vi "DDL.vi"(0 "System no.":i32=1 min=1 max=4 step=1, 2 "Table no.":i32=1, 3 "Offset":i32, 4 "No.of digits":i16=6, 5 "error in":errorcluster, 6 "Values":dbl[](array[numeric]) format="%.6f") -> (19 "error out":errorcluster)   [LabVIEW 2020]
doc: "Loads the specified values to the specified DDL table. Please refer to the controller user manual for units and restrictions.\n\nE-710: Table number can be 1 to 8. First stored value in table has index 1, index 0 must be DDL repeat number. Maximum 32768 values can be stored.\n\nE-712: Table number can be 1 to the maximum number of axes (query with TLT? for the number of DDL tables). First stored value in table has index 1, so Offset must be greater than zero. Maximum 262,144 values can be stored. Due to the maximum numbers of parameters per command only 30 DDL table values can be set per one command call.\n\nE-725, E-727: Table number can be 1 to the maximum number of axes (query with TLT? for the number of DDL tables). First stored value in table has index 1, so Offset must be greater than zero. Maximum 262,144 values can be stored. Due to the maximum numbers of parameters per command only 30 DDL table values can be set per one command call.\n\nE-753: Table number can be 1. First stored value in table has index 1, so Offset must be greater than zero. Maximum 65,536 values can be stored. Due to the maximum numbers of parameters per command only 30 DDL table values can be set per one command call.\n\nE-754: Table number can be 1. First stored value in table has index 1, so Offset must be greater than zero. Maximum 1,046,076 values can be stored. Due to the maximum numbers of parameters per command only 30 DDL table values can be set per one command call."
uses:
  General command.llb/Controller names.ctl
  General command.llb/Global2 (Array).vi
panel:
  # "Loads the specified values to the specified DDL Table. Please refer to \nthe User Manual for units and restrictions."
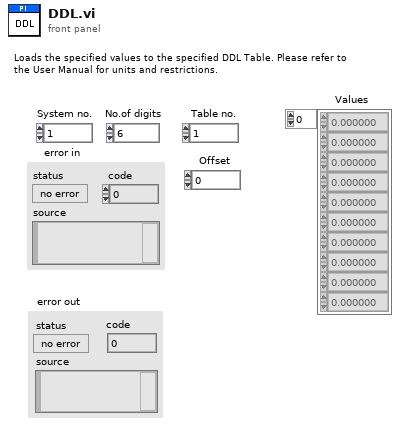
[diagram p1: front panel]
types:
  T1 = typedef "Controller names.ctl" = enum16{"None", "Analog", "C-702", "C-413", "C-414", "C-843", "C-843.PM", "C-844", "C-848", "C-865", "C-866", "C-867", "C-877", "C-880", "C-884", "C-885", "C-886", "C-887", "C-891", "E-135", "E-516", "E-517", "E-518", "E-709", "E-710", "E-712", "E-725", "E-727", "E-753", "E-754", "E-755", "E-761", "E-816", "E-861", "E-870", "E-871", "E-872", "E-873", "E-874", "F-206", "HydraPollux", "M-840", "M-850", "M-8X0", "Mercury", "Mercury_GCS", "PI_GCS2"}
  T2 = cluster{"Conn. axes":string[], "Controller name":T1}[]
  T3 = cluster{"Conn. axes":string[], "Controller name":T1}
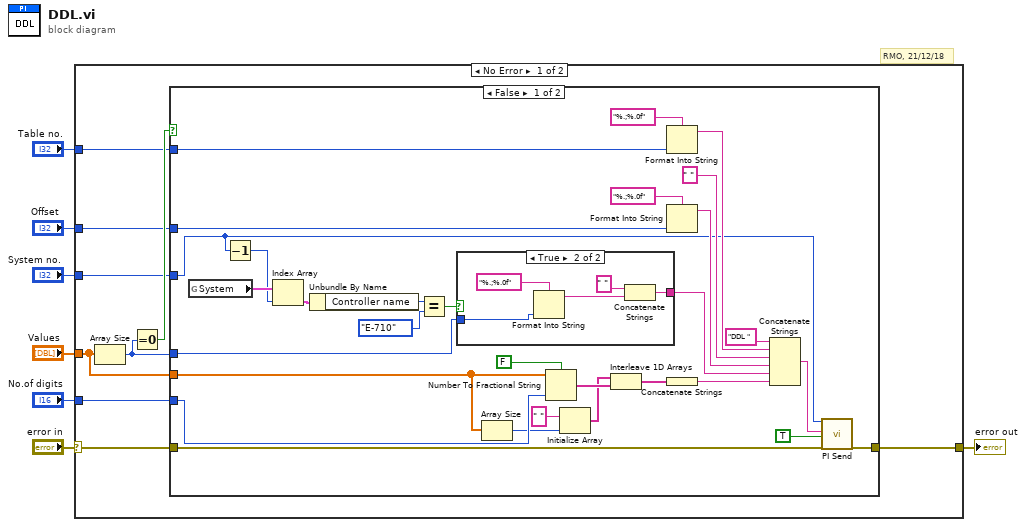
[diagram p0: block diagram]
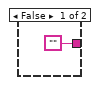
[diagram p2: hidden frame]
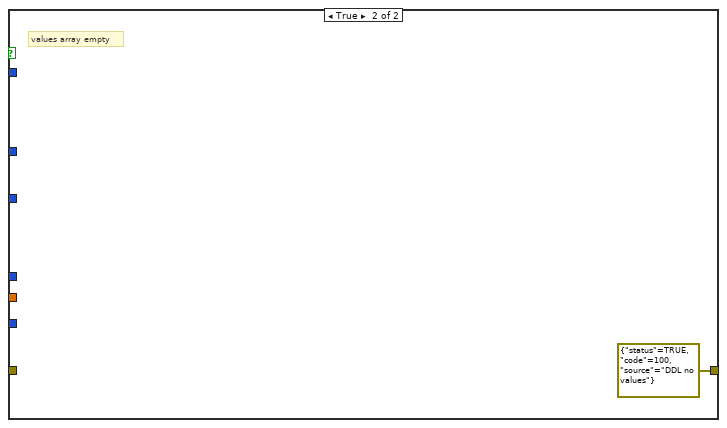
[diagram p3: hidden frame]
diagram:
  # "RMO, 21/12/18"
  n1 = case shown="No Error" "error in" {
    selector: "error in" -> [w13 w54]
    tunnel: [w16 w54] -> w7
    tunnel: "Values" -> [w12 _]
    tunnel: "System no." -> [w11 _]
    tunnel: "Table no." -> [w10 _]
    tunnel: "Offset" -> [w9 _]
    tunnel: "No.of digits" -> [w8 _]
    frame No Error {
      n2 = Array Size(array=w12) -> (size(s)=w14:i32)
      n3 = Equal To 0?(x=w14) -> (x = 0?=w15:bool)
      n4 = case shown="False" w15 {
        tunnel: [w41 errorcluster {"status"=TRUE, "code"=100, "source"="DDL no values"} ("error out")] -> w16
        tunnel: w13 -> [w46 _]
        tunnel: w11 -> [w23 _]
        tunnel: w14 -> [w35 _]
        tunnel: w12 -> [w32 _]
        tunnel: w10 -> [w39 _]
        tunnel: w9 -> [w38 _]
        tunnel: w8 -> [w34 _]
        frame False {
          n5 = global read "Global2 (Array).vi" "System"() -> (w24:T2)
          n6 = Decrement(x=w23) -> (x-1=w22:i32)
          n7 = Index Array(array=w24, index=w22) -> (element=w25:T3)
          n8 = Unbundle By Name(w25) -> ("Controller name"=w21:T1)
          n9 = Equal?(x=w21, y=Controller_names."E-710") -> (x = y?=w19:bool)
          n10 = case shown="True" w19 {
            tunnel: w35 -> [_ w51]
            tunnel: ["" w48] -> w18
            frame False {
            }
            frame True {
              n11 = Format Into String(format string="%.;%.0f" ("Format String"), w51) -> (resulting string=w50:string)  [unwired: 2 in, 1 out]
              n12 = Concatenate Strings(" " ("Substring"), w50) -> (w48:string)
            }
          }
          n13 = Array Size(array=w32) -> (size(s)=w31:i32)
          n14 = Number To Fractional String(use system decimal point (T)=FALSE, number=w32, precision (6)=w34) -> (F-format string=w27:string[])  [unwired: 1 out]
          n15 = Initialize Array(" " ("Element Data"), w31) -> (w26:string[])
          n16 = Interleave 1D Arrays(w26, w27) -> (w29:string[])
          n17 = Format Into String(format string="%.;%.0f" ("Format String"), w39) -> (resulting string=w37:string)  [unwired: 2 in, 1 out]
          n18 = Format Into String(format string="%.;%.0f" ("Format String"), w38) -> (resulting string=w36:string)  [unwired: 2 in, 1 out]
          n19 = Concatenate Strings(w29) -> (w17:string)
          n20 = Concatenate Strings("DDL ", w37, " " ("Substring"), w36, w18, w17) -> (w42:string)
          n21 = call "PI Send.vi"("System no."=w23, "String to send"=w42, "Attach termination char.?"=TRUE ("Attach Linefeed?"), "error in"=w46) -> ("error out"=w41:errorcluster)  [unwired: 2 in, 13 out]
        }
        frame True {
          # "values array empty"
        }
      }
    }
    frame Error {
    }
  }
  "error out" <- w7
